vi "pid_test.vi"() -> ()   [LabVIEW 2019]
uses:
  <vilib>/addons/control/pid/NI_PID_autopid.lvlib
panel:
  out "tuning completed?":bool
  out "Waveform Chart":dbl(graph)
  out "XY Graph":cluster{dbl[], dbl[]}[](graph)
  in  "stop":bool
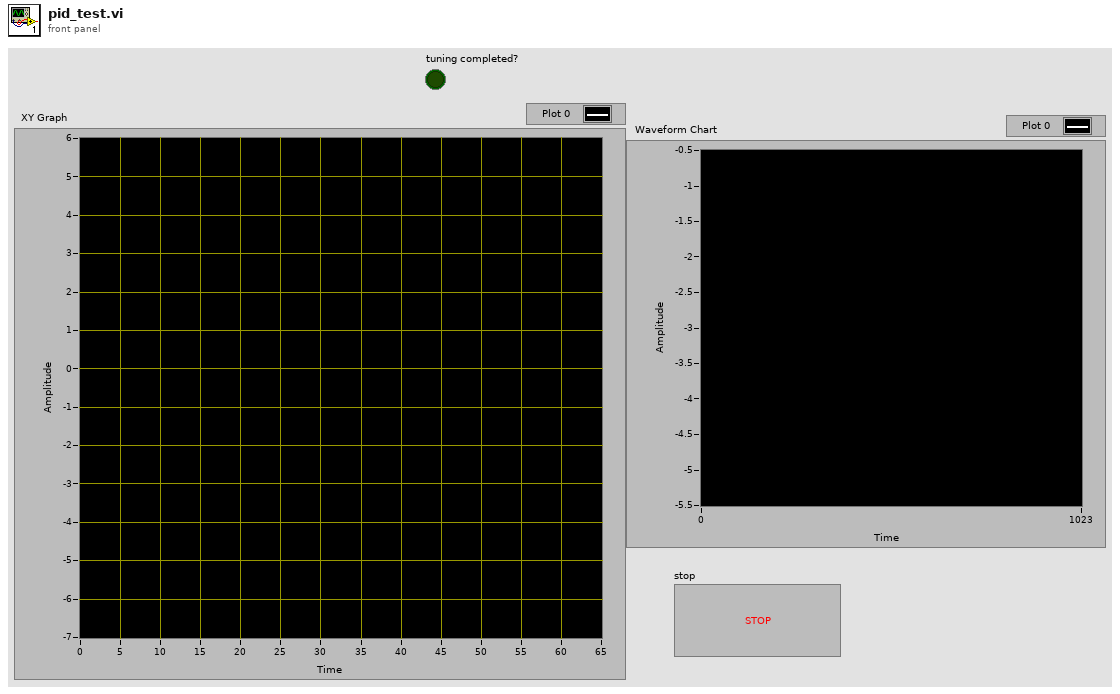
[diagram p1: front panel]
types:
  T1 = cluster{"controller type":u16, "relay cycles":i32, "relay amplitude":dbl, "control specification":u16, "PV noise level":dbl}
  T2 = cluster{"proportional gain (Kc)":dbl, "integral time (Ti, min)":dbl, "derivative time (Td, min)":dbl}
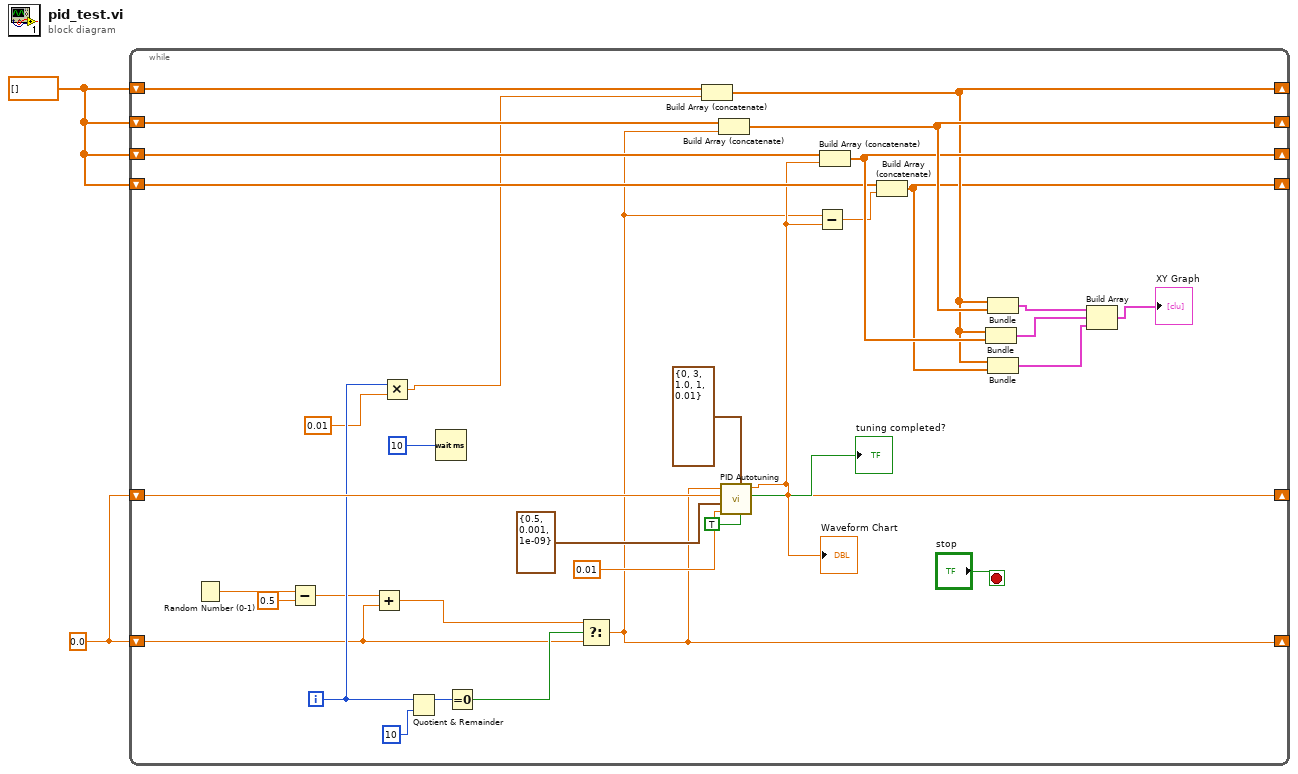
[diagram p0: block diagram]
diagram:
  w1 = dbl[] []
  w2 = 0.0 ("dt (s)")
  n1 = while {
    shift-right: [w13] -> _
    shift-left: w1 -> [w35]
    shift-right: [w32] -> _
    shift-left: w1 -> [w34]
    shift-right: [w28] -> _
    shift-left: w1 -> [w33]
    shift-right: [w15] -> _
    shift-left: w2 -> [w3]
    shift-right: [w16] -> _
    shift-left: w2 -> [w17]
    shift-right: [w12] -> _
    shift-left: w1 -> [w18]
    i -> [w10]
    stop <- "stop" stop-if-true
    n2 = Random Number (0-1)() -> (number: 0 to 1=w6:dbl)
    n3 = Subtract(x=w6, y=0.5) -> (x-y=w4:dbl)
    n4 = Add(x=w4, y=w3) -> (x+y=w7:dbl)
    n5 = Multiply(x=w10, y=0.01 ("x")) -> (x*y=w8:dbl)
    n6 = Quotient & Remainder(x=w10, y=10) -> (x-y*floor(x/y)=w26:i32)  [unwired: 1 out]
    n7 = Wait (ms)(milliseconds to wait=u32 10) -> ()  [unwired: 1 out]
    n8 = Equal To 0?(x=w26) -> (x = 0?=w25:bool)
    n9 = Select(t=w7, s=w25, f=w3) -> (s? t:f=w15:dbl)
    n10 = Build Array (concatenate)(w35, w8) -> (w13:dbl[])
    n11 = Build Array (concatenate)(w34, w15) -> (w32:dbl[])
    n12 = call <vilib>:"PID Autotuning.vi"("autotune? (F)"=TRUE, "autotuning parameters"=T1 {"controller type"=0, "relay cycles"=3, "relay amplitude"=1.0, "control specification"=1, "PV noise level"=0.01}, "dt (s)"=0.01, "PID gains"=T2 {"proportional gain (Kc)"=0.5, "integral time (Ti, min)"=0.001, "derivative time (Td, min)"=1e-09}, "process variable"=w17, "setpoint"=w15) -> ("tuning completed?"=→"tuning completed?":bool, "output"=w16:dbl)  [unwired: 2 in, 2 out]
    "Waveform Chart" <- w16
    n13 = Subtract(x=w15, y=w16) -> (x-y=w14:dbl)
    n14 = Build Array (concatenate)(w33, w16) -> (w28:dbl[])
    n15 = Build Array (concatenate)(w18, w14) -> (w12:dbl[])
    n16 = Bundle(w13, w28) -> (w29:cluster{dbl[], dbl[]})  [unwired: 1 in]
    n17 = Bundle(w13, w32) -> (w31:cluster{dbl[], dbl[]})  [unwired: 1 in]
    n18 = Bundle(w13, w12) -> (w11:cluster{dbl[], dbl[]})  [unwired: 1 in]
    n19 = Build Array(w31, w29, w11) -> (→"XY Graph":cluster{dbl[], dbl[]}[])
  }
